vi "Agilent ENA Series Interactive Application.vi"() -> ()   [LabVIEW 2020]
doc: "Illustrates typical measuring task for a network analyzer. The described measured task is transmission measurement of magnitude and phase."
uses:
  <instrlib>/Agilent ENA Series/Agilent ENA Series.lvlib
panel:
  in  "Save State (F: Disable)":bool
  out "High":dbl
  out "Low":dbl
  out "Center Frequency":dbl format="%^.2e"
  out "Q Value":dbl format="%^.2e"
  out "Loss":dbl format="%^.2e"
  out "Bandwidth":dbl format="%^.2e"
  in  "Power (dBm)":dbl=-10.0 format="%^.2e"
  in  "IF Bandwidth":dbl=10000.0 format="%^.2e"
  in  "Span Frequency [Hz]":dbl=200000000.0 format="%^.2e"
  in  "Center Frequency [Hz]":dbl=947500000.0 format="%^.2e"
  in  "VISA resource name":refnum<visa-resource-name>
  # "(c) 2005-2021 National Instruments.  ALL RIGHTS RESERVED."
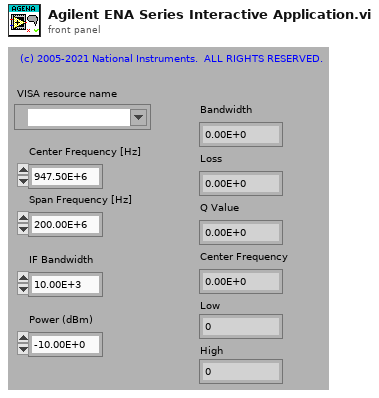
[diagram p1: front panel]
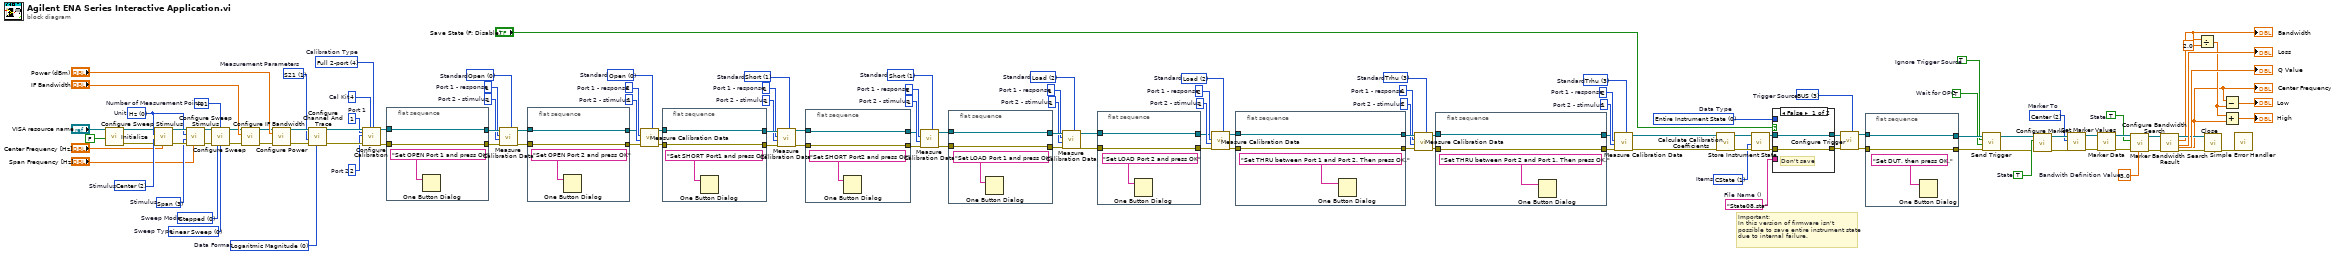
[diagram p0: block diagram]
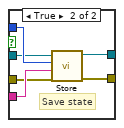
[diagram p2: hidden frame]
diagram:
  w34 = -3.0  # Bandwith Definition Value
  w35 = TRUE  # State
  w40 = u16 2 items=["Start", "Stop", "Center", "Reference", "Electrical Delay"]  # Marker To
  w43 = TRUE  # State
  w44 = TRUE  # Wait for OPC
  w45 = TRUE  # Ignore Trigger Source
  w50 = u16 3 items=["Internal", "External", "Manual", "BUS"]  # Trigger Source
  w16 = "State08.sta"  # File Name ()
  w17 = u16 0 items=["Entire Instrument State", "Formatted Data Array", "Image On The LCD Display", "Segment Sweep Table", "Limit Table", "Power Sensor A", "Power Sensor B", "VBA Project", "Loss Compensation Table 1", "Loss Compensation Table 2", "Loss Compensation Table 3", "Loss Compensation Table 4"]  # Data Type
  w1 = u16 1 items=["State", "CState", "Dstate", "CDState"]  # Items
  w53 = u16 3 items=["Open", "Short", "Load", "Trhu", "Isolation"]  # Standard
  w55 = 1  # Port 2 - stimulus
  w54 = 2  # Port 1 - response
  w62 = u16 3 items=["Open", "Short", "Load", "Trhu", "Isolation"]  # Standard
  w58 = 2  # Port 2 - stimulus
  w59 = 1  # Port 1 - response
  w65 = u16 2 items=["Open", "Short", "Load", "Trhu", "Isolation"]  # Standard
  w69 = 1  # Port 2 - stimulus
  w68 = 2  # Port 1 - response
  w76 = u16 2 items=["Open", "Short", "Load", "Trhu", "Isolation"]  # Standard
  w72 = 1  # Port 2 - stimulus
  w73 = 1  # Port 1 - response
  w79 = u16 1 items=["Open", "Short", "Load", "Trhu", "Isolation"]  # Standard
  w83 = 1  # Port 2 - stimulus
  w82 = 2  # Port 1 - response
  w90 = u16 1 items=["Open", "Short", "Load", "Trhu", "Isolation"]  # Standard
  w86 = 1  # Port 2 - stimulus
  w87 = 1  # Port 1 - response
  w91 = u16 0 items=["Open", "Short", "Load", "Trhu", "Isolation"]  # Standard
  w92 = u16 0 items=["Open", "Short", "Load", "Trhu", "Isolation"]  # Standard
  w98 = 1  # Port 2 - stimulus
  w97 = 2  # Port 1 - response
  w99 = 1  # Port 2 - stimulus
  w100 = 1  # Port 1 - response
  w105 = 2  # Port 2
  w106 = 1  # Port 1
  w107 = u16 4 items=["Open", "Short", "Through", "1-port", "Full 2-port", "Full 3-port", "Full 4-port"]  # Calibration Type
  w108 = 4  # Cal Kit
  w111 = u16 0 items=["Logaritmic Magnitude", "Phase", "Group Delay", "Smith Chart  Linear (Lin/Phase)", "Smith Chart  Logaritmic (Log/Phase)", "Smith Chart  Complex (Real/Imag)", "Smith Chart  Impedance (R+jX)", "Smith Chart  Admittance (G+jB)", "Polar Format (Linear)", "Polar Format (Logaritmic)", "Polar Format (Re/Im)", "Linear Magnitude", "SWR", "Real", "Imaginary", "Epanded Phase", "Positive Phase"]  # Data Format
  w112 = u16 1 items=["S11", "S21", "S31", "S41", "S12", "S22", "S32", "S42", "S13", "S23", "S33", "S43", "S14", "S24", "S34", "S44", "A", "B", "C", "D", "R1", "R2", "R3", "R4"]  # Measurement Parameters
  w123 = u16 0 items=["Linear Sweep", "Logaritmic Sweep", "Segment Sweep", "Power Sweep"]  # Sweep Type
  w124 = 401  # Number of Measurement Points
  w125 = u16 0 items=["Stepped", "Swept", "Fast Stepped Mode", "Fast Swept Mode"]  # Sweep Mode
  w128 = u16 3 items=["Start", "Stop", "Center", "Span"]  # Stimulus
  w126 = u16 0 items=["Hz", "kHz", "MHz", "GHz", "dBm", "s"]  # Unit
  w132 = u16 2 items=["Start", "Stop", "Center", "Span"]  # Stimulus
  # "Important:\nIn this version of firmware isn't \npossible to save entire instrument state\ndue to internal failure."
  n1 = call <instrlib>:"Initialize.vi"("Reset? (T: Yes)"=FALSE, "VISA resource name"="VISA resource name") -> ("error out"=w18:errorcluster, "VISA resource name out"=w19:refnum<visa-resource-name>)  [unwired: 8 in]
  n2 = call <instrlib>:"Configure Sweep Stimulus.vi"("Parameter (0.0)"="Center Frequency [Hz]", "error in (no error)"=w18, "Stimulus (0: Start)"=w132, "Unit (0: Hz)"=w126, "VISA resource name"=w19) -> ("error out"=w130:errorcluster, "VISA resource name out"=w129:refnum<visa-resource-name>)  [unwired: 5 in]
  n3 = call <instrlib>:"Configure Sweep Stimulus.vi"("Parameter (0.0)"="Span Frequency [Hz]", "error in (no error)"=w130, "Stimulus (0: Start)"=w128, "Unit (0: Hz)"=w126, "VISA resource name"=w129) -> ("error out"=w122:errorcluster, "VISA resource name out"=w121:refnum<visa-resource-name>)  [unwired: 5 in]
  n4 = call <instrlib>:"Configure Sweep.vi"("VISA resource name"=w121, "Number of Measurement Points (201)"=w124, "error in (no error)"=w122, "Sweep Mode (0: Stepped)"=w125, "Sweep Type (0: Linear Sweep)"=w123) -> ("VISA resource name out"=w119:refnum<visa-resource-name>, "error out"=w118:errorcluster)  [unwired: 9 in]
  n5 = call <instrlib>:"Configure IF Bandwidth.vi"("error in (no error)"=w118, "IF Bandwidth (100000.0)"="IF Bandwidth", "VISA resource name"=w119) -> ("error out"=w116:errorcluster, "VISA resource name out"=w115:refnum<visa-resource-name>)  [unwired: 7 in]
  n6 = call <instrlib>:"Configure Power.vi"("VISA resource name"=w115, "Power Level (0.0)"="Power (dBm)", "error in (no error)"=w116) -> ("VISA resource name out"=w114:refnum<visa-resource-name>, "error out"=w113:errorcluster)  [unwired: 11 in]
  n7 = call <instrlib>:"Configure Channel And Trace.vi"("Data Format (0: Logarithmic Magnitude)"=w111, "error in (no error)"=w113, "Measurement Parameters (0: S11)"=w112, "VISA resource name"=w114) -> ("error out"=w109:errorcluster, "VISA resource name out"=w110:refnum<visa-resource-name>)  [unwired: 6 in]
  n8 = call <instrlib>:"Configure Calibration.vi"("VISA resource name"=w110, "Port 1 (1)"=w106, "Port 2 (1)"=w105, "error in (no error)"=w109, "Cal Kit (1)"=w108, "Calibration Type (6: Full 4-port)"=w107) -> ("VISA resource name out"=w104:refnum<visa-resource-name>, "error out"=w103:errorcluster)  [unwired: 12 in]
  n9 = flat-sequence {
    tunnel: w104 -> [w134]
    tunnel: w103 -> [w133]
    tunnel: [w133] -> w101
    tunnel: [w134] -> w102
    frame #0 {
      n10 = One Button Dialog(message="Set OPEN Port 1 and press OK") -> ()  [unwired: 1 in, 1 out]
    }
  }
  n11 = call <instrlib>:"Measure Calibration Data.vi"("Standard (0: Open)"=w92, "error in (no error)"=w101, "Port 2 - stimulus (2)"=w99, "Port 1 - response (1)"=w100, "VISA resource name"=w102) -> ("error out"=w93:errorcluster, "VISA resource name out"=w94:refnum<visa-resource-name>)  [unwired: 5 in]
  n12 = flat-sequence {
    tunnel: w94 -> [w137]
    tunnel: w93 -> [w136]
    tunnel: [w136] -> w96
    tunnel: [w137] -> w95
    frame #0 {
      n13 = One Button Dialog(message="Set OPEN Port 2 and press OK") -> ()  [unwired: 1 in, 1 out]
    }
  }
  n14 = call <instrlib>:"Measure Calibration Data.vi"("Standard (0: Open)"=w91, "error in (no error)"=w96, "Port 2 - stimulus (2)"=w98, "Port 1 - response (1)"=w97, "VISA resource name"=w95) -> ("error out"=w84:errorcluster, "VISA resource name out"=w85:refnum<visa-resource-name>)  [unwired: 5 in]
  n15 = flat-sequence {
    tunnel: w85 -> [w140]
    tunnel: w84 -> [w139]
    tunnel: [w139] -> w88
    tunnel: [w140] -> w89
    frame #0 {
      n16 = One Button Dialog(message="Set SHORT Port1 and press OK") -> ()  [unwired: 1 in, 1 out]
    }
  }
  n17 = call <instrlib>:"Measure Calibration Data.vi"("Standard (0: Open)"=w90, "error in (no error)"=w88, "Port 2 - stimulus (2)"=w86, "Port 1 - response (1)"=w87, "VISA resource name"=w89) -> ("error out"=w77:errorcluster, "VISA resource name out"=w78:refnum<visa-resource-name>)  [unwired: 5 in]
  n18 = flat-sequence {
    tunnel: w78 -> [w143]
    tunnel: w77 -> [w142]
    tunnel: [w142] -> w81
    tunnel: [w143] -> w80
    frame #0 {
      n19 = One Button Dialog(message="Set SHORT Port2 and press OK") -> ()  [unwired: 1 in, 1 out]
    }
  }
  n20 = call <instrlib>:"Measure Calibration Data.vi"("Standard (0: Open)"=w79, "error in (no error)"=w81, "Port 2 - stimulus (2)"=w83, "Port 1 - response (1)"=w82, "VISA resource name"=w80) -> ("error out"=w70:errorcluster, "VISA resource name out"=w71:refnum<visa-resource-name>)  [unwired: 5 in]
  n21 = flat-sequence {
    tunnel: w71 -> [w146]
    tunnel: w70 -> [w145]
    tunnel: [w145] -> w74
    tunnel: [w146] -> w75
    frame #0 {
      n22 = One Button Dialog(message="Set LOAD Port 1 and press OK") -> ()  [unwired: 1 in, 1 out]
    }
  }
  n23 = call <instrlib>:"Measure Calibration Data.vi"("Standard (0: Open)"=w76, "error in (no error)"=w74, "Port 2 - stimulus (2)"=w72, "Port 1 - response (1)"=w73, "VISA resource name"=w75) -> ("error out"=w63:errorcluster, "VISA resource name out"=w64:refnum<visa-resource-name>)  [unwired: 5 in]
  n24 = flat-sequence {
    tunnel: w64 -> [w149]
    tunnel: w63 -> [w148]
    tunnel: [w148] -> w67
    tunnel: [w149] -> w66
    frame #0 {
      n25 = One Button Dialog(message="Set LOAD Port 2 and press OK") -> ()  [unwired: 1 in, 1 out]
    }
  }
  n26 = call <instrlib>:"Measure Calibration Data.vi"("Standard (0: Open)"=w65, "error in (no error)"=w67, "Port 2 - stimulus (2)"=w69, "Port 1 - response (1)"=w68, "VISA resource name"=w66) -> ("error out"=w56:errorcluster, "VISA resource name out"=w57:refnum<visa-resource-name>)  [unwired: 5 in]
  n27 = flat-sequence {
    tunnel: w57 -> [w152]
    tunnel: w56 -> [w151]
    tunnel: [w151] -> w60
    tunnel: [w152] -> w61
    frame #0 {
      n28 = One Button Dialog(message="Set THRU between Port 1 and Port 2. Then press OK.") -> ()  [unwired: 1 in, 1 out]
    }
  }
  n29 = call <instrlib>:"Measure Calibration Data.vi"("Standard (0: Open)"=w62, "error in (no error)"=w60, "Port 2 - stimulus (2)"=w58, "Port 1 - response (1)"=w59, "VISA resource name"=w61) -> ("error out"=w51:errorcluster, "VISA resource name out"=w52:refnum<visa-resource-name>)  [unwired: 5 in]
  n30 = flat-sequence {
    tunnel: w52 -> [w155]
    tunnel: w51 -> [w154]
    tunnel: [w154] -> w9
    tunnel: [w155] -> w10
    frame #0 {
      n31 = One Button Dialog(message="Set THRU between Port 2 and Port 1. Then press OK.") -> ()  [unwired: 1 in, 1 out]
    }
  }
  n32 = call <instrlib>:"Measure Calibration Data.vi"("Standard (0: Open)"=w53, "error in (no error)"=w9, "Port 2 - stimulus (2)"=w55, "Port 1 - response (1)"=w54, "VISA resource name"=w10) -> ("error out"=w6:errorcluster, "VISA resource name out"=w7:refnum<visa-resource-name>)  [unwired: 5 in]
  n33 = call <instrlib>:"Calculate Calibration Coefficients.vi"("error in (no error)"=w6, "VISA resource name"=w7) -> ("error out"=w5:errorcluster, "VISA resource name out"=w4:refnum<visa-resource-name>)  [unwired: 8 in]
  n34 = call <instrlib>:"Store Instrument State.vi"("error in (no error)"=w5, "Items (3: CDState)"=w1, "VISA resource name"=w4) -> ("error out"=w2:errorcluster, "VISA resource name out"=w3:refnum<visa-resource-name>)  [unwired: 7 in]
  n35 = case shown="False" "Save State (F: Disable)" {
    tunnel: w17 -> [_ w164]
    tunnel: w16 -> [_ w163]
    tunnel: w3 -> [w158 w162]
    tunnel: [w158 w161] -> w15
    tunnel: w2 -> [w157 w160]
    tunnel: [w157 w159] -> w14
    frame False {
      # "Don't save"
    }
    frame True {
      # "Save state"
      n36 = call <instrlib>:"Store.vi"("error in (no error)"=w160, "File Name ()"=w163, "Data Type (0: Entire Instrument State)"=w164, "VISA resource name"=w162) -> ("error out"=w159:errorcluster, "VISA resource name out"=w161:refnum<visa-resource-name>)  [unwired: 6 in]
    }
  }
  n37 = call <instrlib>:"Configure Trigger.vi"("Trigger Source (0: Internal)"=w50, "error in (no error)"=w14, "VISA resource name"=w15) -> ("error out"=w48:errorcluster, "VISA resource name out"=w49:refnum<visa-resource-name>)  [unwired: 7 in]
  n38 = flat-sequence {
    tunnel: w49 -> [w165]
    tunnel: w48 -> [w166]
    tunnel: [w166] -> w46
    tunnel: [w165] -> w47
    frame #0 {
      n39 = One Button Dialog(message="Set DUT, then press OK.") -> ()  [unwired: 1 in, 1 out]
    }
  }
  n40 = call <instrlib>:"Send Trigger.vi"("error in (no error)"=w46, "Wait for OPC (F: Do not Wait)"=w44, "Ignore Trigger Source (F: Do not Ignore)"=w45, "VISA resource name"=w47) -> ("error out"=w11:errorcluster, "VISA resource name out"=w12:refnum<visa-resource-name>)  [unwired: 6 in]
  n41 = call <instrlib>:"Configure Marker.vi"("error in (no error)"=w11, "Marker State (F: Disabled)"=w43, "VISA resource name"=w12) -> ("error out"=w41:errorcluster, "VISA resource name out"=w42:refnum<visa-resource-name>)  [unwired: 7 in]
  n42 = call <instrlib>:"Set Marker Values.vi"("error in (no error)"=w41, "Marker To (0: Start)"=w40, "VISA resource name"=w42) -> ("error out"=w38:errorcluster, "VISA resource name out"=w39:refnum<visa-resource-name>)  [unwired: 7 in]
  n43 = call <instrlib>:"Marker Data.vi"("error in (no error)"=w38, "VISA resource name"=w39) -> ("error out"=w36:errorcluster, "VISA resource name out"=w37:refnum<visa-resource-name>)  [unwired: 5 in, 3 out]
  n44 = call <instrlib>:"Configure Bandwidth Search.vi"("Bandwidth Definition Value (-3.0)"=w34, "error in (no error)"=w36, "Result Display State (F: Disable)"=w35, "VISA resource name"=w37) -> ("error out"=w32:errorcluster, "VISA resource name out"=w33:refnum<visa-resource-name>)  [unwired: 6 in]
  n45 = call <instrlib>:"Marker Bandwidth Search Result.vi"("error in (no error)"=w32, "VISA resource name"=w33) -> ("error out"=w28:errorcluster, "Loss"=→"Loss":dbl, "Bandwidth"=w27:dbl, "VISA resource name out"=w29:refnum<visa-resource-name>, "Q Value"=→"Q Value":dbl, "Center Frequency"=w23:dbl)  [unwired: 4 in]
  "Bandwidth" <- w27
  "Center Frequency" <- w23
  n46 = Divide(x=w27, y=2.0) -> (x/y=w24:dbl)
  n47 = call <instrlib>:"Close.vi"("error in (no error)"=w28, "VISA resource name"=w29) -> ("error out"=w21:errorcluster)  [unwired: 9 in]
  n48 = Subtract(x=w23, y=w24) -> (x-y=→"Low":dbl)
  n49 = Add(x=w24, y=w23) -> (x+y=→"High":dbl)
  n50 = call <vilib>:"Simple Error Handler.vi"("error in (no error)"=w21) -> ()  [unwired: 4 in, 5 out]
